vi "recorder.vi"() -> ()   [LabVIEW 2015]
panel:
  out "Next":string="Bence\n\n"
  in  "Elotag":string="M11_"
  out "Recording on":bool
  in  "Stop Button":bool
  # "M11 F15"
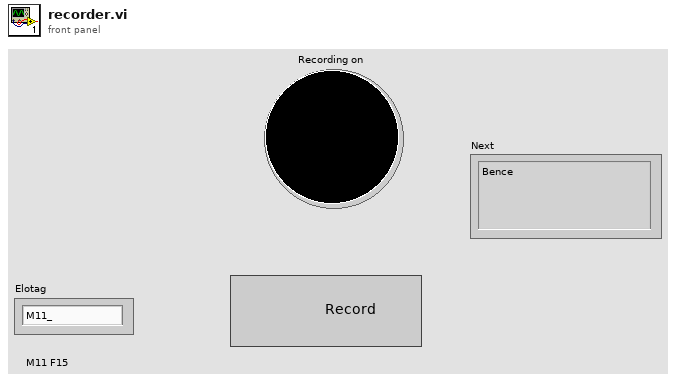
[diagram p1: front panel]
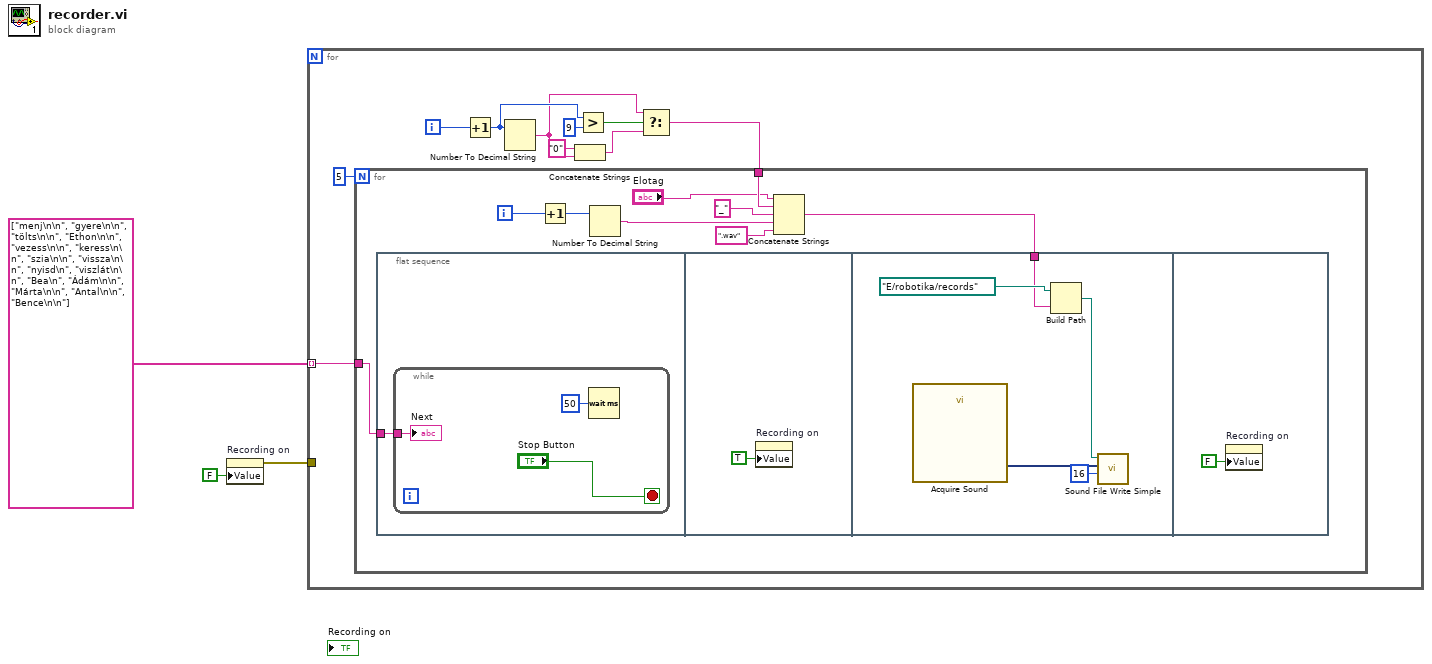
[diagram p0: block diagram]
diagram:
  n1 = property on="Recording on" class="Bool (strict)"("Value"=FALSE ("Recording on")) -> (error out=w2:errorcluster)  [unwired: 2 in, 1 out]
  n2 = for {
    tunnel: w2 -> [_]
    tunnel: string[] ["menj\n\n", "gyere\n\n", "tölts\n\n", "Ethon\n\n", "vezess\n\n", "keress\n\n", "szia\n\n", "vissza\n\n", "nyisd\n", "viszlát\n\n", "Bea\n", "Ádám\n\n", "Márta\n\n", "Antal\n\n", "Bence\n\n"] -> [w13] mode=indexing
    i -> [w12]
    n3 = Increment(x=w12) -> (x+1=w10:i32)
    n4 = Number To Decimal String(number=w10) -> (decimal integer string=w5:string)  [unwired: 1 in]
    n5 = Concatenate Strings("0" ("string"), w5) -> (w7:string)
    n6 = Greater?(x=w10, y=9) -> (0:w8:bool)
    n7 = Select(t=w5, s=w8, f=w7) -> (s? t:f=w4:string)
    n8 = for {
      N: 5 -> [_]
      tunnel: w13 -> [w16]
      tunnel: w4 -> [w20]
      i -> [w22]
      n9 = flat-sequence {
        tunnel: w16 -> [w23]
        tunnel: w17 -> [w29]
        frame #0 {
          n10 = while {
            tunnel: w23 -> [w24]
            stop <- "Stop Button" stop-if-true
            n11 = Wait (ms)(milliseconds to wait=u32 50) -> ()  [unwired: 1 out]
            "Next" <- w24
          }
        }
        frame #1 {
          n12 = property on="Recording on" class="Bool (strict)"("Value"=TRUE ("Recording on")) -> ()  [unwired: 2 in, 2 out]
        }
        frame #2 {
          n13 = call "Acquire Sound"() -> ("Data"=w32:dynamicdata)  [unwired: 18 in, 1 out]
          n14 = Build Path(base path=path "E:/robotika/records" ("path"), name or relative path=w29) -> (appended path=w28:path)
          n15 = call <vilib>:"Sound File Write Simple.vi"("bits per sample"=16, "data"=w32, "path"=w28) -> ()  [unwired: 7 in, 2 out]
        }
        frame #3 {
          n16 = property on="Recording on" class="Bool (strict)"("Value"=FALSE ("Recording on")) -> ()  [unwired: 2 in, 2 out]
        }
      }
      n17 = Increment(x=w22) -> (x+1=w21:i32)
      n18 = Number To Decimal String(number=w21) -> (decimal integer string=w19:string)  [unwired: 1 in]
      n19 = Concatenate Strings("Elotag", w20, "_" ("string"), w19, ".wav" ("string")) -> (w17:string)
    }
  }
